vi "GetNoOfTrials&TrialsUsed(SubVI).vi"(10 "Admin no":string, 11 "Refnum in":T1) -> (1 "NoOfTrialsUsed":i32, 3 "NoOfTrials":i32)   [LabVIEW 2013]
uses:
  <vilib>/addons/database/Connection.llb/Conn ObjectReference.ctl
  <vilib>/addons/database/_DB Variant To Data/Database Variant To Data.xnode
  <vilib>/addons/database/NI_Database_API.lvlib
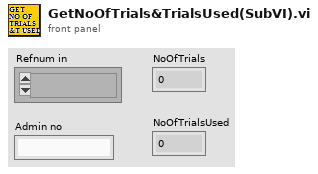
[diagram p1: front panel]
types:
  T1 = typedef "NI_Database_API.lvlib/Conn ObjectReference.ctl" = refnum<k1>
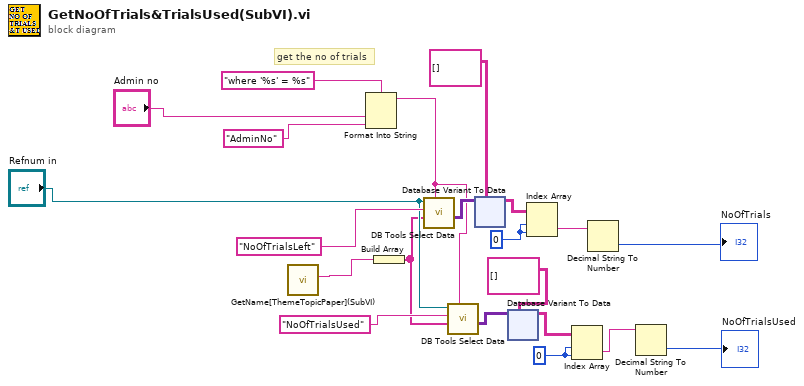
[diagram p0: block diagram]
diagram:
  w3 = 0 ("disabled index (col)")
  w15 = 0 ("disabled index (col)")
  # "get the no of trials"
  n1 = call "GetName[ThemeTopicPaper](SubVI).vi"() -> ("Path for Score Table"=w19:string)  [unwired: 11 in]
  n2 = Format Into String(format string="where '%s' = %s", "Admin no", "AdminNo") -> (resulting string=w7:string)  [unwired: 2 in, 1 out]
  n3 = Build Array(w19) -> (w8:string[])
  n4 = call <vilib>:"DB Tools Select Data.vi"("condition"=w7, "columns"=w8, "table"="NoOfTrialsLeft", "connection reference"="Refnum in") -> ("data"=w16:variant[][])  [unwired: 2 in, 2 out]
  n5 = call <vilib>:"DB Tools Select Data.vi"("condition"=w7, "columns"=w8, "table"="NoOfTrialsUsed", "connection reference"="Refnum in") -> ("data"=w6:variant[][])  [unwired: 2 in, 2 out]
  n6 = xnode "Database Variant To Data"("database variant"=w16, "type"=string[][] []) -> ("data"=w18:string[][])  [unwired: 1 in, 1 out]
  n7 = xnode "Database Variant To Data"("database variant"=w6, "type"=string[][] []) -> ("data"=w4:string[][])  [unwired: 1 in, 1 out]
  n8 = Index Array(array=w18, index (row)=w15, index (col)=w15) -> (element=w14:string)
  n9 = Index Array(array=w4, index (row)=w3, index (col)=w3) -> (element=w2:string)
  n10 = Decimal String To Number(string=w14) -> (number=→"NoOfTrials":i32)  [unwired: 2 in, 1 out]
  n11 = Decimal String To Number(string=w2) -> (number=→"NoOfTrialsUsed":i32)  [unwired: 2 in, 1 out]
